vi "main.vi"() -> ()   [LabVIEW 2021]
uses:
  D:/Common/LabVIEW GEA2 Toolkit/source/GEA3 DLL Source/GeaCommunication.dll
  Common/LabVIEW GEA2 Toolkit/source/GEA3 DLL Source/GeaCommunication.dll
panel:
  in  "Ticket Name":string
  out "Data Result":T1(array[cluster])
  out "Version":T2
  in  "Board Index":u8 max=1 step=1
  # "0901"
  # "pos 11"
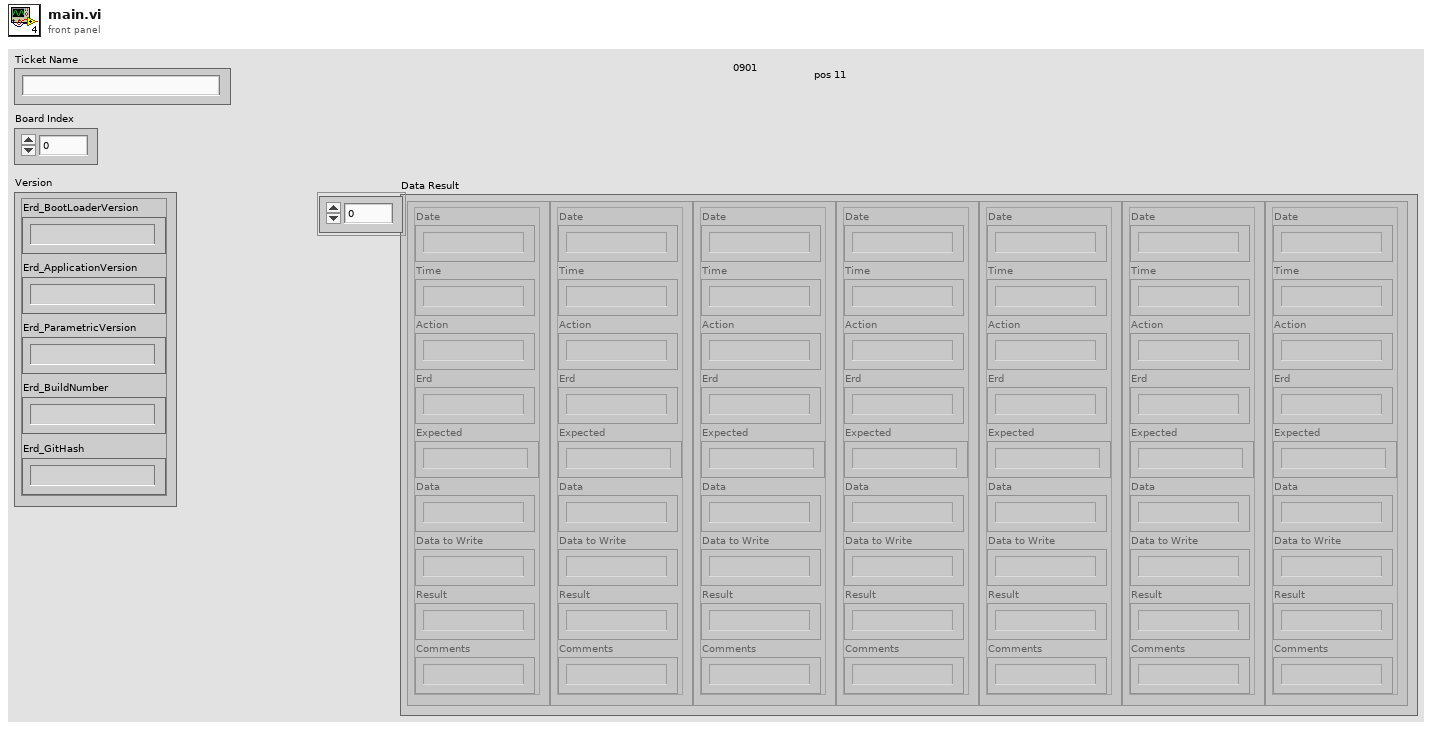
[diagram p1: front panel]
types:
  T1 = cluster{"Date":string, "Time":string, "Action":string, "Erd":string, "Expected":string, "Data":string, "Data to Write":string, "Result":string, "Comments":string}[]
  T2 = cluster{"Erd_BootLoaderVersion":string, "Erd_ApplicationVersion":string, "Erd_ParametricVersion":string, "Erd_BuildNumber":string, "Erd_GitHash":string}
  T3 = cluster{"dst":string, "ACTION":string, "ERD":string, "Expected":string, "WriteDato":string}[]
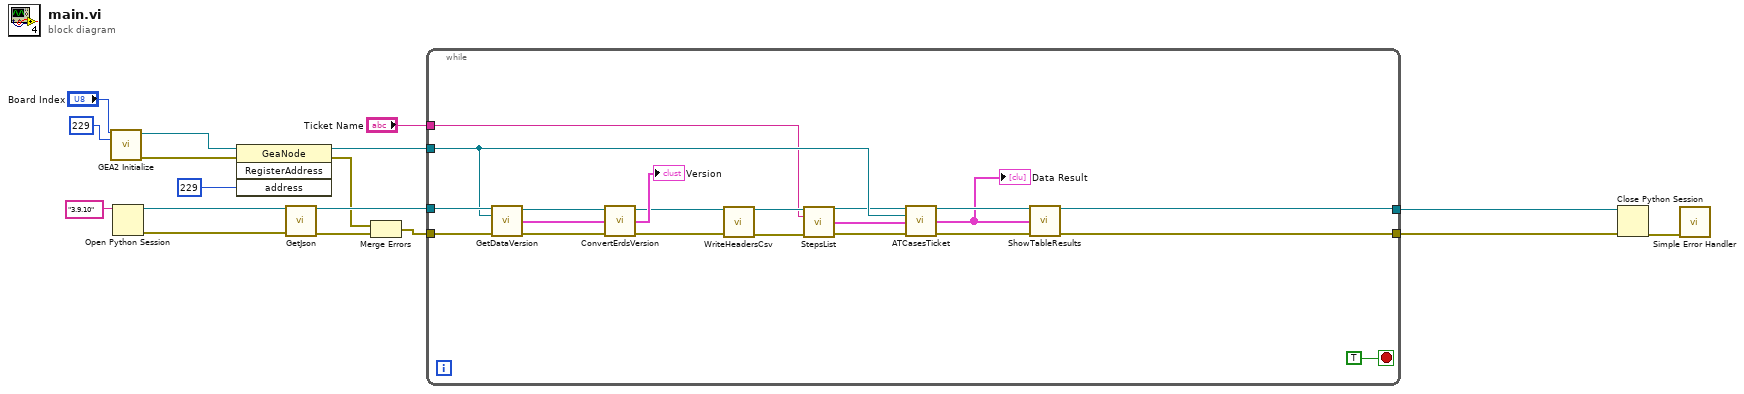
[diagram p0: block diagram]
diagram:
  n1 = call "GEA2 Initialize.vi"("Board Index"="Board Index", "Source Address"=u8 229) -> ("GEA2 Reference Out"=w15:refnum<k24>, "error out"=w14:errorcluster)  [unwired: 11 in, 1 out]
  n2 = Open Python Session(python version="3.9.10" ("Python version")) -> (session out=w10:refnum<k35>, error out=w9:errorcluster)  [unwired: 2 in]
  n3 = invoke class="GeaNode" method="RegisterAddress"(reference=w15, error in=w14, "address"=u8 229 ("Source Address")) -> (reference out=w6:refnum<k24>, error out=w3:errorcluster)  [unwired: 1 in, 2 out]
  n4 = call "GetJson.vi"("session in"=w10, "error in"=w9) -> ("session out"=w5:refnum<k35>, "error out"=w4:errorcluster)  [unwired: 12 in]
  n5 = Merge Errors(w3, w4) -> (w8:errorcluster)
  n6 = while {
    tunnel: w6 -> [w27]
    tunnel: w8 -> [w35]
    tunnel: [w22] -> w11
    tunnel: [w21] -> w7
    tunnel: w5 -> [w28]
    tunnel: "Ticket Name" -> [w18]
    stop <- TRUE stop-if-true
    n7 = call "GetDataVersion.vi"("session In"=w28, "GEA2 Reference In"=w27, "error In"=w35) -> ("session out"=w30:refnum<k35>, "Data Version Out"=w34:cluster{"ERD Number":u16, "Data":string}[], "error out"=w26:errorcluster)  [unwired: 10 in]
    n8 = call "ConvertErdsVersion.vi"("Erds_Version"=w34, "error in"=w26) -> ("Version out"=→"Version":T2, "error out"=w25:errorcluster)  [unwired: 12 in]
    n9 = call "WriteHeadersCsv.vi"("session in"=w30, "error in"=w25) -> ("session out"=w31:refnum<k35>, "error out"=w32:errorcluster)  [unwired: 12 in]
    n10 = call "StepsList.vi"("session in"=w31, "Ticket Name"=w18, "error in"=w32) -> ("session out"=w24:refnum<k35>, "return value"=w29:T3, "error out"=w20:errorcluster)  [unwired: 10 in]
    n11 = call "ATCasesTicket.vi"("session in"=w24, "GEA2 Reference In"=w27, "Steps"=w29) -> ("session out"=w23:refnum<k35>, "Data Result"=w19:T1)  [unwired: 10 in, 1 out]
    "Data Result" <- w19
    n12 = call "ShowTableResults.vi"("session in"=w23, "Data Result"=w19, "error in"=w20) -> ("session out"=w22:refnum<k35>, "error out"=w21:errorcluster)  [unwired: 11 in]
  }
  n13 = Close Python Session(session in=w11, error in=w7) -> (11:w2:errorcluster)
  n14 = call <vilib>:"Simple Error Handler.vi"("error in (no error)"=w2) -> ()  [unwired: 4 in, 5 out]
